vi "getColorFromDocument.vi"(8 "error in (no error)":errorcluster, 11 "xwpfRun in":refnum<class "xwpfRun.lvclass">) -> (0 "error out":errorcluster, 3 "xwpfRun out":refnum<class "xwpfRun.lvclass">)   [LabVIEW 2017, in "Word_Specific.lvlib" / "xwpfRun.lvclass"]
uses:
  xwpfRun.lvclass
  xwpfRun.lvclass/xwpfRun.ctl
  C:/Users/Neo/Desktop/Dev_Tools_BR/LabVIEW_NPOI/src/lib/NPOI 2.1.1/NPOI.OOXML.dll
  lib/NPOI 2.1.1/NPOI.OOXML.dll
  Styles/Style/Style.lvclass
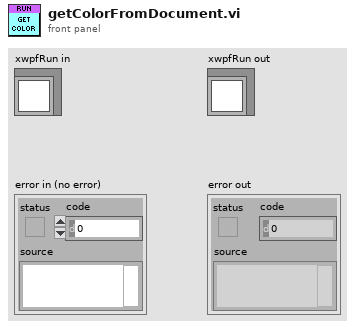
[diagram p1: front panel]
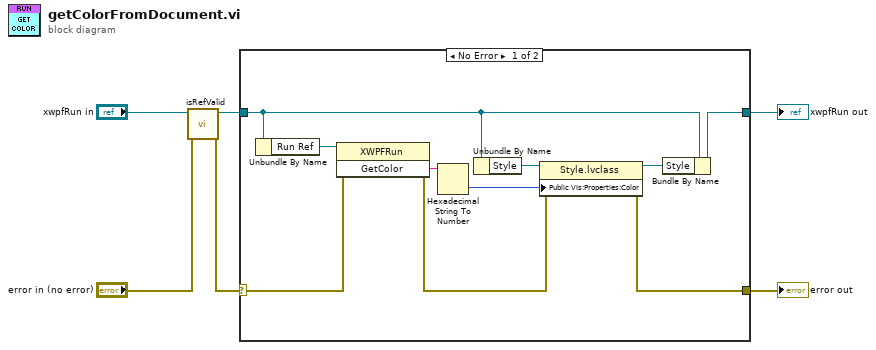
[diagram p0: block diagram]
diagram:
  n1 = call-dynamic "isRefValid.vi"("error in (no error)"="error in (no error)", "xwpfRun in"="xwpfRun in") -> ("error out"=w1:errorcluster, "xwpfRun out"=w3:refnum<class "xwpfRun.lvclass">)  [unwired: 8 in]
  n2 = case shown="No Error" w1 {
    selector: w1 -> [w16 w18]
    tunnel: [w14 w18] -> w6
    tunnel: [w15 w17] -> w4
    tunnel: w3 -> [w13 w17]
    frame No Error {
      n3 = Unbundle By Name(w13) -> ("Run Ref"=w12:refnum<k24>)
      n4 = invoke class="XWPFRun" method="GetColor"(reference=w12, error in=w16) -> (error out=w7:errorcluster, "GetColor"=w11:string)  [unwired: 1 in, 1 out]
      n5 = Hexadecimal String To Number(string=w11) -> (number=w8:u32)  [unwired: 2 in, 1 out]
      n6 = Unbundle By Name(w13) -> ("Style"=w10:refnum<class "Style.lvclass">)
      n7 = property class="Style.lvclass"(reference=w10, error in=w7, "Public VIs:Properties:Color"=w8) -> (reference out=w9:refnum<class "Style.lvclass">, error out=w14:errorcluster)
      n8 = Bundle By Name(cluster=w13, "Style"=w9) -> (w15:refnum<class "xwpfRun.lvclass">)
    }
    frame Error {
    }
  }
  "error out" <- w6
  "xwpfRun out" <- w4
